vi "ConvertScanSizeto01.vi"(8 "error in (no error)":errorcluster, 9 "Parameters In":T1={"fastRoundPts"=32, "slowRoundPts"=8, "fastWaveType"=enum."Rounded", "slowWaveType"=enum."Triangle", "fastWavePts"=1024, "slowWavePts"=1024, "outputRateHz"=800000, "yOffset"=0.0, "xOffset"=0.0, "scanSizeSlow"=0.5, "scanSizeFast"=0.5, "rotation"=0.0, "timePerLine"=0.01, "numLines"=256, "pointsPerLine"=512, "scanEnable"=FALSE, "slowMoveWavePts"=1024, "slowMoveAccelPts"=128, "moveSpeedSec"=0.2, "singleDirectionScan"=FALSE} {"yOffset" min=0.0 max=1.0 format="%#_6p"; "xOffset" min=0.0 max=1.0 format="%#_6p"; "scanSizeSlow" min=0.0 max=1.0 format="%#_6p"; "scanSizeFast" min=0.0 max=1.0 format="%#_6p"; "timePerLine" min=0.001 max=100.0 format="%#_6p"; "outputRateHz" format="%.0p"}, 10 "Calibration":cluster{"Slow":dbl, "Fast":dbl, "Z":dbl}={"Slow"=0.00015, "Fast"=0.00015, "Z"=0.00015}) -> (0 "error out":errorcluster, 1 "Parameters Out":T1={"fastRoundPts"=32, "slowRoundPts"=8, "fastWaveType"=enum."Rounded", "slowWaveType"=enum."Triangle", "fastWavePts"=1024, "slowWavePts"=1024, "outputRateHz"=800000, "yOffset"=0.0, "xOffset"=0.0, "scanSizeSlow"=0.5, "scanSizeFast"=0.5, "rotation"=0.0, "timePerLine"=0.01, "numLines"=256, "pointsPerLine"=512, "scanEnable"=FALSE, "slowMoveWavePts"=1024, "slowMoveAccelPts"=128, "moveSpeedSec"=0.2, "singleDirectionScan"=FALSE} {"yOffset" min=0.0 max=1.0 format="%#_6p"; "xOffset" min=0.0 max=1.0 format="%#_6p"; "scanSizeSlow" min=0.0 max=1.0 format="%#_6p"; "scanSizeFast" min=0.0 max=1.0 format="%#_6p"; "timePerLine" min=0.001 max=100.0 format="%#_6p"; "outputRateHz" format="%.0p"}, 2 "Slow":dbl=0.00015, 3 "Fast":dbl=0.00015, 4 "Z":dbl=0.00015)   [LabVIEW 2016]
uses:
  FGV/ScanParametersAllTypeDef.ctl
  controls/ScanWaveform.ctl
panel:
  # "scanWaveFormCtl"
  # "slowMoveParameters"
  # "scanCtl"
  # "ioParams"
  # "scanWaveFormCtl"
  # "slowMoveParameters"
  # "scanCtl"
  # "ioParams"
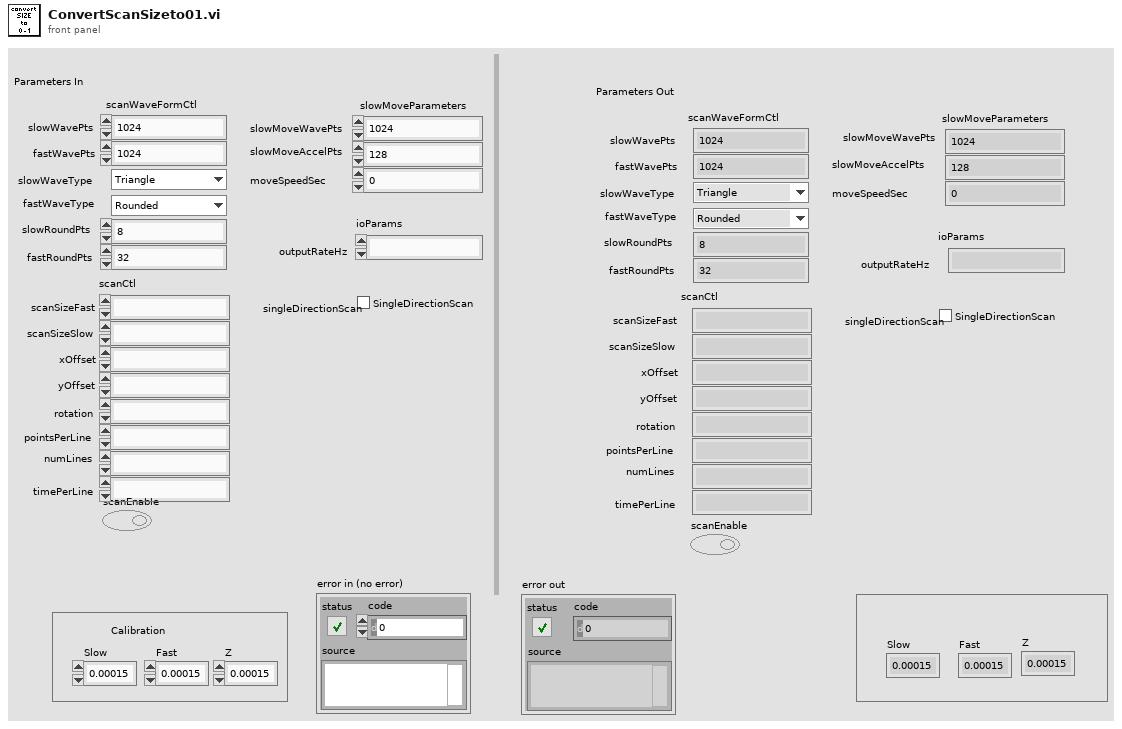
[diagram p1: front panel]
types:
  T1 = typedef "ScanParametersAllTypeDef.ctl" = cluster{"fastRoundPts":u16, "slowRoundPts":u16, "fastWaveType":T2, "slowWaveType":T2, "fastWavePts":u16, "slowWavePts":u16, "outputRateHz":u32, "yOffset":dbl, "xOffset":dbl, "scanSizeSlow":dbl, "scanSizeFast":dbl, "rotation":dbl, "timePerLine":dbl, "numLines":u16, "pointsPerLine":u32, "scanEnable":bool, "slowMoveWavePts":u16, "slowMoveAccelPts":u16, "moveSpeedSec":dbl, "singleDirectionScan":bool}
  T2 = typedef "ScanWaveform.ctl" = enum16{"Sine", "Triangle", "Rounded"}
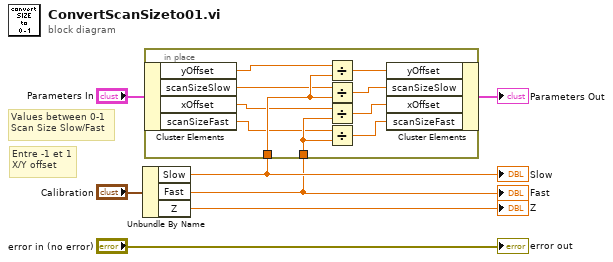
[diagram p0: block diagram]
diagram:
  # "Entre -1 et 1\nX/Y offset"
  # "Values between 0-1\nScan Size Slow/Fast"
  n1 = Unbundle By Name("Calibration") -> ("Slow"=w5:dbl, "Fast"=w4:dbl, "Z"=→"Z":dbl)
  "Slow" <- w5
  "Fast" <- w4
  n2 = in-place {
    in-place-border: w5 -> [w17]
    in-place-border: w4 -> [w16]
    n3 = in-place-cluster #1("Parameters In") -> ("yOffset"=w15:dbl, "scanSizeSlow"=w13:dbl, "xOffset"=w11:dbl, "scanSizeFast"=w9:dbl)
    n4 = Divide(x=w15, y=w17) -> (x/y=w14:dbl)
    n5 = Divide(x=w13, y=w17) -> (x/y=w12:dbl)
    n6 = Divide(x=w11, y=w16) -> (x/y=w10:dbl)
    n7 = Divide(x=w9, y=w16) -> (x/y=w8:dbl)
    n8 = in-place-cluster #1("yOffset"=w14, "scanSizeSlow"=w12, "xOffset"=w10, "scanSizeFast"=w8) -> (→"Parameters Out":T1)
  }
  "error out" <- "error in (no error)"
